vi "Lookup Log Channel Index.vi"(6 "Exact Value (T)":bool=TRUE, 8 "error in (no error)":errorcluster, 9 "Meta Value":string, 10 "Config Element in":refnum<class "Config Element.lvclass">, 11 "Group in":refnum<class "Group DBL.lvclass">) -> (0 "error out":errorcluster, 1 "Index":i32, 2 "Config Element":refnum<class "Config Element.lvclass">, 3 "Group":refnum<class "Group DBL.lvclass">)   [LabVIEW 2020, in "VolatusData.lvlib" / "Log Manager Module.lvclass"]
uses:
  Log Manager Module.lvclass
  lv-cdm/CDM-Config/Config Element/Config Element.lvclass
  lv-vecto/Vecto/Group DBL/Group DBL.lvclass
  C:/dev/lv20CE/relink/lv-vecto/Vecto/Group/Group.lvclass
  lv-cdm/CDM-Config/Config Element/Owner.vi
  lv-cdm/CDM-Config/Config Manager/Lookup Descendant.vi
  lv-vecto/Vecto/Group/Group.lvclass
  lv-cdm/CDM-Config/Config Filter/Config Lookup.lvclass
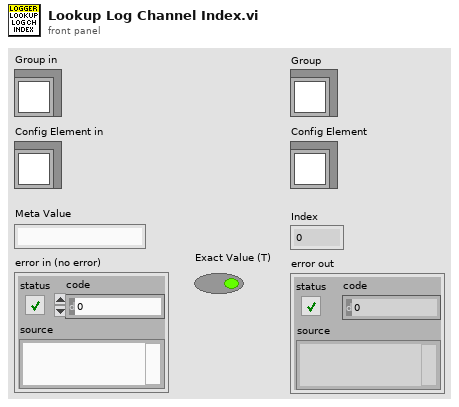
[diagram p1: front panel]
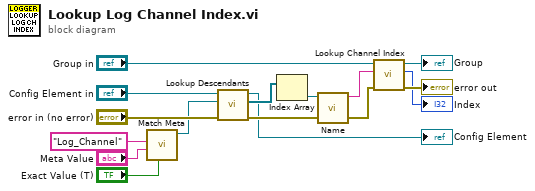
[diagram p0: block diagram]
diagram:
  n1 = call "Match Meta.vi"("Exact Value (F)"="Exact Value (T)", "Value (Any)"="Meta Value", "Name"="Log_Channel") -> ("Config Lookup out"=w9:refnum<class "Config Lookup.lvclass">)  [unwired: 7 in, 1 out]
  n2 = call "Lookup Descendants.vi"("error in (no error)"="error in (no error)", "Lookup"=w9, "Config Element in"="Config Element in") -> ("error out"=w4:errorcluster, "Descendants"=w12:refnum<class "Config Element.lvclass">[], "Config Element out"=→"Config Element":refnum<class "Config Element.lvclass">)  [unwired: 6 in]
  n3 = Index Array(array=w12) -> (element=w11:refnum<class "Config Element.lvclass">)  [unwired: 1 in]
  n4 = call "Name.vi"("Config Element in"=w11) -> ("Name"=w8:string)  [unwired: 9 in, 1 out]
  n5 = call "Lookup Channel Index.vi"("error in (no error)"=w4, "Channel Name"=w8, "GroupAbstract in"="Group in") -> ("error out"=→"error out":errorcluster, "Index"=→"Index":i32, "GroupAbstract out"=→"Group":refnum<class "Group DBL.lvclass">)  [unwired: 6 in]
